vi "Queue FGV.vi"(7 "FGV States":T1, 8 "error in":errorcluster, 11 "Queue Name":string) -> (0 "error out":errorcluster, 3 "queue out":refnum<queue>)   [LabVIEW 2024, in "QMH Messaging.lvlib"]
uses:
  QMH Messaging.lvlib
  General Type Defs/FGV States.ctl
  General Type Defs/Queue Message.ctl
  General Type Defs/General Type Defs.lvlib
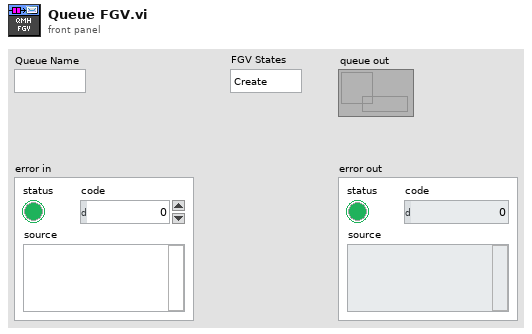
[diagram p1: front panel]
types:
  T1 = typedef "General Type Defs.lvlib/FGV States.ctl" = enum16{"Create", "Get", "Destroy"}
  T2 = typedef "General Type Defs.lvlib/Queue Message.ctl" = cluster{"Message":string, "Value":variant}
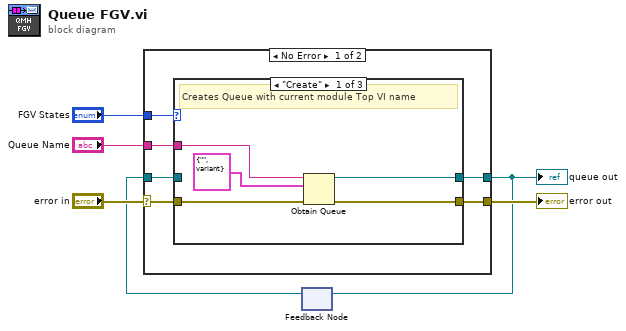
[diagram p0: block diagram]
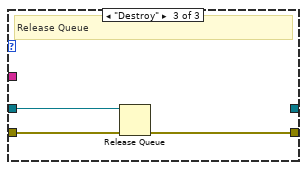
[diagram p3: hidden frame]
diagram:
  n1 = feedback #1() -> (w2:refnum<queue>)  [unwired: 1 in]
  n2 = case shown="No Error" "error in" {
    selector: "error in" -> [w9 w23]
    tunnel: "FGV States" -> [w12 _]
    tunnel: [w11 w23] -> w5
    tunnel: "Queue Name" -> [w10 _]
    tunnel: [w8 _] -> w1
    tunnel: w2 -> [w7 _]
    frame No Error {
      n3 = case shown="\"Create\"" w12 {
        tunnel: [w17 w18 w21] -> w11
        tunnel: w9 -> [w16 w18 w22]
        tunnel: w10 -> [w14 _ _]
        tunnel: [w13 w19 _] -> w8
        tunnel: w7 -> [_ w19 w20]
        frame "Create" {
          # "Creates Queue with current module Top VI name"
          n4 = Obtain Queue(name (unnamed)=w14, element data type=T2 {"Message"="", "Value"=variant}, error in (no error)=w16) -> (queue out=w13:refnum<queue>, error out=w17:errorcluster)  [unwired: 2 in, 1 out]
        }
        frame "Get", Default {
          # "Gets Queue"
        }
        frame "Destroy" {
          # "Release Queue"
          n5 = Release Queue(queue=w20, error in (no error)=w22) -> (error out=w21:errorcluster)  [unwired: 1 in, 2 out]
        }
      }
    }
    frame Error {
    }
  }
  "error out" <- w5
  "queue out" <- w1
  n6 = feedback-in #1(w1) -> ()
